vi "Execute.vi"(8 "error in":errorcluster, 9 "Consumer Queues in":T1, 10 "DAC Process Command in":refnum<class "Start DAC.lvclass">, 11 "DAC Process Data in":T2) -> (0 "error out":errorcluster, 1 "Consumer Queues out":T1, 2 "Stop?":bool, 3 "DAC Process Data out":T2)   [LabVIEW 2019, in "DAC Process.lvlib" / "Start DAC.lvclass"]
uses:
  Start DAC.lvclass
  Generic Test Stand/Generic Test Stand.lvclass
  Generic DAC Command/Generic DAC Process Command.lvclass
  Generic Test Stand/TS Panel Method.ctl
  Trig Process/TRIG Next Acq Request/TRIG Next Acq Request.lvclass
  DAC Process Data.ctl
  DAC Process.lvlib
  UI Process/Generic UI Command/Generic UI Process Command.lvclass
  TS Framework/Consumer Queues.ctl
  TS Framework/TS Framework.lvlib
  TS Framework/ExeLogging/DAC Logger/DAC Logger.lvclass
  DAC State.ctl
  Trig Process/Generic Trig Command/Generic Trig Process Command.lvclass
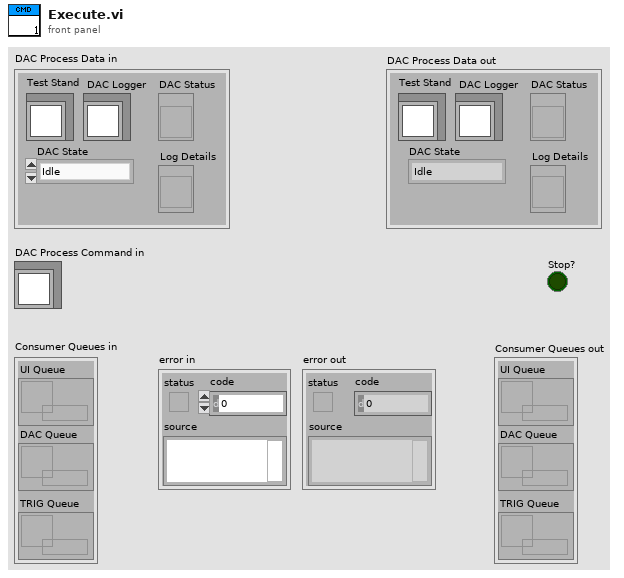
[diagram p1: front panel]
types:
  T1 = typedef "TS Framework.lvlib/Consumer Queues.ctl" = cluster{"UI Queue":refnum<queue>, "DAC Queue":refnum<queue>, "TRIG Queue":refnum<queue>}
  T2 = typedef "DAC Process.lvlib/DAC Process Data.ctl" = cluster{"Test Stand":refnum<class "Generic Test Stand.lvclass">, " DAC Logger":refnum<class "DAC Logger.lvclass">, "DAC State":T3, "DAC Status":refnum<vi>, "Log Details":refnum<vi>}
  T3 = typedef "DAC Process.lvlib/DAC State.ctl" = enum16{"Idle", "Acquiring"}
  T4 = typedef "Generic Test Stand.lvclass/TS Panel Method.ctl" = enum16{"Send to Panel", "Receive from Panel", "Update Panel View"}
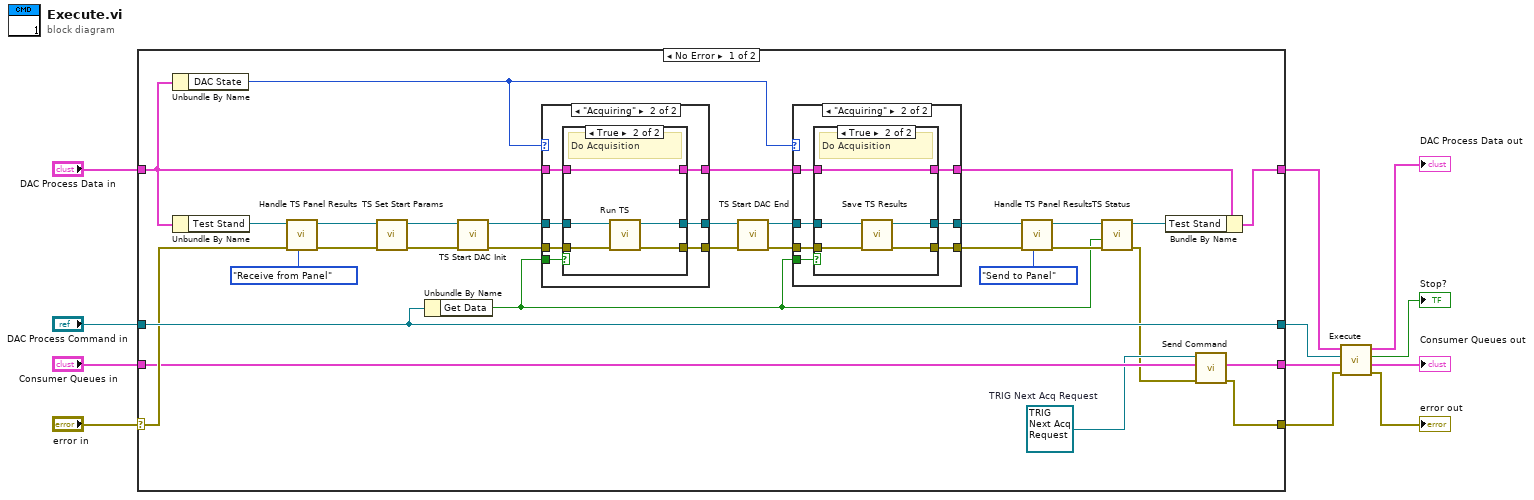
[diagram p0: block diagram]
diagram:
  n1 = case shown="No Error" "error in" {
    selector: "error in" -> [w31 w83]
    tunnel: [w21 w83] -> w7
    tunnel: "Consumer Queues in" -> [w25 w82]
    tunnel: [w24 w82] -> w5
    tunnel: "DAC Process Data in" -> [w43 w81]
    tunnel: [w40 w81] -> w3
    tunnel: "DAC Process Command in" -> [w34 w80]
    tunnel: [w34 w80] -> w1
    frame No Error {
      w23 = refnum<class "TRIG Next Acq Request.lvclass"> refnum  # TRIG Next Acq Request
      n2 = Unbundle By Name(w43) -> ("DAC State"=w13:T3)
      n3 = Unbundle By Name(w43) -> ("Test Stand"=w29:refnum<class "Generic Test Stand.lvclass">)
      n4 = call-dynamic "Handle TS Panel Results.vi"("Method"=TS_Panel_Method."Receive from Panel", "error in"=w31, "Test Stand in"=w29) -> ("error out"=w30:errorcluster, "Test Stand out"=w28:refnum<class "Generic Test Stand.lvclass">)  [unwired: 7 in]
      n5 = call-dynamic "TS Set Start Params.vi"("error in (no error)"=w30, "Generic Test Stand in"=w28) -> ("error out"=w35:errorcluster, "Generic Test Stand out"=w36:refnum<class "Generic Test Stand.lvclass">)  [unwired: 8 in]
      n6 = Unbundle By Name(w34) -> ("Get Data"=w14:bool)
      n7 = call-dynamic "TS Start DAC Init.vi"("error in"=w35, "Test Stand in"=w36) -> ("error out"=w39:errorcluster, "Test Stand out"=w42:refnum<class "Generic Test Stand.lvclass">)  [unwired: 8 in]
      n8 = case shown="\"Acquiring\"" w13 {
        tunnel: w43 -> [w64 w71]
        tunnel: [w64 w70] -> w20
        tunnel: w42 -> [w63 w69]
        tunnel: [w63 w68] -> w41
        tunnel: w14 -> [_ w67]
        tunnel: w39 -> [w62 w66]
        tunnel: [w62 w65] -> w38
        frame "Idle", Default {
        }
        frame "Acquiring" {
          n9 = case shown="True" w67 {
            tunnel: w71 -> [w74 w79]
            tunnel: [w74 w79] -> w70
            tunnel: w69 -> [w73 w78]
            tunnel: [w73 w76] -> w68
            tunnel: w66 -> [w72 w77]
            tunnel: [w72 w75] -> w65
            frame False {
              # "Do Not Acquisition"
            }
            frame True {
              # "Do Acquisition"
              n10 = call-dynamic "Run TS.vi"("error in"=w77, "Test Stand in"=w78) -> ("error out"=w75:errorcluster, "Test Stand out"=w76:refnum<class "Generic Test Stand.lvclass">)  [unwired: 8 in]
            }
          }
        }
      }
      n11 = call-dynamic "TS Start DAC End.vi"("error in"=w38, "Test Stand in"=w41) -> ("error out"=w18:errorcluster, "Test Stand out"=w19:refnum<class "Generic Test Stand.lvclass">)  [unwired: 8 in]
      n12 = case shown="\"Acquiring\"" w13 {
        tunnel: w20 -> [w46 w53]
        tunnel: [w46 w52] -> w17
        tunnel: w19 -> [w45 w51]
        tunnel: [w45 w50] -> w16
        tunnel: w14 -> [_ w49]
        tunnel: w18 -> [w44 w48]
        tunnel: [w44 w47] -> w15
        frame "Idle", Default {
        }
        frame "Acquiring" {
          n13 = case shown="True" w49 {
            tunnel: w53 -> [w56 w61]
            tunnel: [w56 w61] -> w52
            tunnel: w51 -> [w55 w58]
            tunnel: [w55 w60] -> w50
            tunnel: w48 -> [w54 w57]
            tunnel: [w54 w59] -> w47
            frame False {
              # "Do Not Acquisition"
            }
            frame True {
              # "Do Acquisition"
              n14 = call-dynamic "Save TS Results.vi"("error in"=w57, "Test Stand in"=w58) -> ("error out"=w59:errorcluster, "Test Stand out"=w60:refnum<class "Generic Test Stand.lvclass">)  [unwired: 8 in]
            }
          }
        }
      }
      n15 = call-dynamic "Handle TS Panel Results.vi"("Method"=TS_Panel_Method."Send to Panel", "error in"=w15, "Test Stand in"=w16) -> ("error out"=w26:errorcluster, "Test Stand out"=w27:refnum<class "Generic Test Stand.lvclass">)  [unwired: 7 in]
      n16 = call-dynamic "TS Status.vi"("error in"=w26, "New Data?"=w14, "Test Stand in"=w27) -> ("error out"=w22:errorcluster, "Test Stand out"=w37:refnum<class "Generic Test Stand.lvclass">)  [unwired: 7 in]
      n17 = Bundle By Name(cluster=w17, "Test Stand"=w37) -> (w40:T2)
      n18 = call-dynamic "Send Command.vi"("error in (no error)"=w22, "Consumer Queues in"=w25, "Trig Process Command"=w23) -> ("error out"=w21:errorcluster, "Consumer Queues out"=w24:T1)  [unwired: 7 in]
    }
    frame Error {
    }
  }
  n19 = call-parent "Execute.vi"("error in"=w7, "Consumer Queues in"=w5, "DAC Process Command in"=w1, "DAC Process Data in"=w3) -> ("error out"=→"error out":errorcluster, "Consumer Queues out"=→"Consumer Queues out":T1, "Stop?"=→"Stop?":bool, "DAC Process Data out"=→"DAC Process Data out":T2)  [unwired: 4 in]
